vi "Global Settings.vi"() -> ()   [LabVIEW 2019, in "Configuration Tool.lvlib"]
uses:
  Configuration Tool.lvlib
panel:
  in  "VeriStand Version (String)":string
  in  "Target Project Ref":refnum<vi>
  in  "Target Project Name":string(combo)
  in  "VeriStand Version":enum16{"2013", "2014", "2015", "2016"}(ring)=enum."2015"
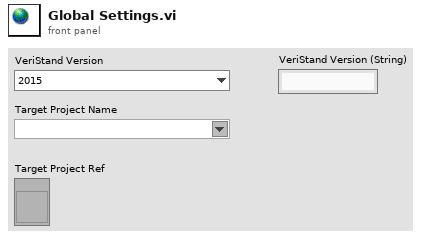
[diagram p1: front panel]
diagram:
